vi "Get ni_measurementlink_measurement_v1_GetMetadataResponse.vi"(8 "error in (no error)":errorcluster, 11 "gRPCid":T1) -> (0 "error out":errorcluster, 2 "package_templatemessage":T2, 3 "gRPCid out":T1)   [LabVIEW 2020, in "MeasurementLink Measurement Server Internal.lvlib"]
uses:
  MeasurementLink Measurement Server Internal.lvlib
  ni_measurementlink_measurement_v1_GetMetadataResponse.ctl
  ni_measurementlink_measurement_v1_MeasurementDetails.ctl
  ni_measurementlink_measurement_v1_MeasurementSignature.ctl
  ni_measurementlink_measurement_v1_ConfigurationParameter.ctl
  google_protobuf_Field_Kind.ctl
  ni_measurementlink_measurement_v1_ConfigurationParameter_AnnotationsEntry.ctl
  google_protobuf_Any.ctl
  ni_measurementlink_measurement_v1_Output.ctl
  ni_measurementlink_measurement_v1_UserInterfaceDetails.ctl
  <vilib>/gRPC/LabVIEW gRPC Library/Shared/grpcId.ctl
  ni_measurementlink_measurement_v1_GetMetadataResponse_Flat.ctl
  ni_measurementlink_measurement_v1_MeasurementDetails_Flat.ctl
  ni_measurementlink_measurement_v1_MeasurementSignature_Flat.ctl
  ni_measurementlink_measurement_v1_ConfigurationParameter_Flat.ctl
  ni_measurementlink_measurement_v1_ConfigurationParameter_AnnotationsEntry_Flat.ctl
  google_protobuf_Any_Flat.ctl
  ni_measurementlink_measurement_v1_Output_Flat.ctl
  ni_measurementlink_measurement_v1_UserInterfaceDetails_Flat.ctl
  2ed25e12-861d-4677-8ead-ace2906b2041.vi
  <vilib>/gRPC/LabVIEW gRPC Library/Shared/TranslateGrpcError.vi
  FlatToRichni_measurementlink_measurement_v1_MeasurementDetails.vi
  FlatToRichni_measurementlink_measurement_v1_MeasurementSignature.vi
  FlatToRichni_measurementlink_measurement_v1_UserInterfaceDetails.vi
  FlatToRichni_measurementlink_measurement_v1_ConfigurationParameter.vi
  FlatToRichgoogle_protobuf_Any.vi
  FlatToRichni_measurementlink_measurement_v1_Output.vi
  FlatToRichni_measurementlink_measurement_v1_ConfigurationParameter_AnnotationsEntry.vi
  <vilib>/gRPC/LabVIEW gRPC Library/Server API/Server/Get Server DLL Path.vi
  <vilib>/Utility/error.llb/Error Cluster From Error Code.vi
  <vilib>/Utility/error.llb/Simple Error Handler.vi
  <vilib>/gRPC/LabVIEW gRPC Library/grpc-lvsupport-release.lvlib
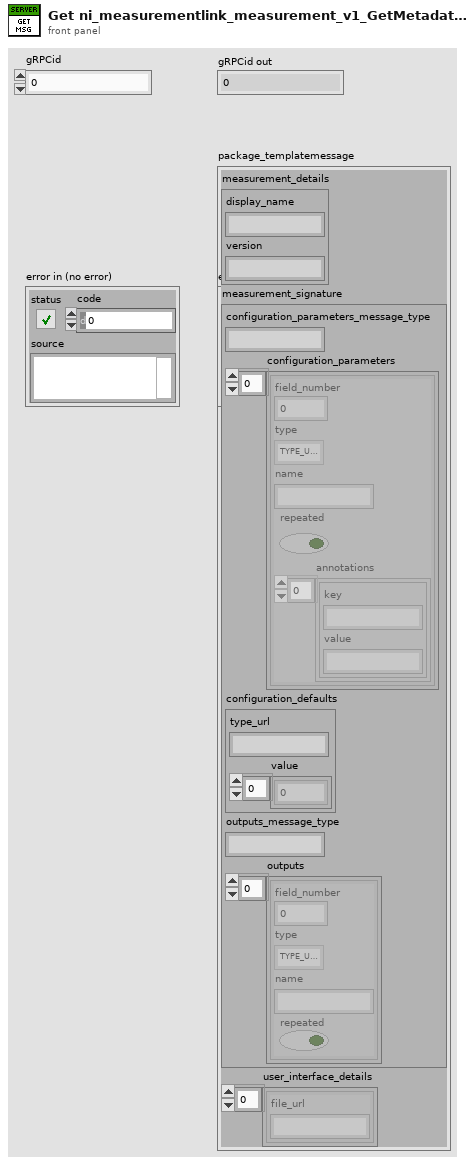
[diagram p1: front panel]
types:
  T1 = typedef "grpc-lvsupport-release.lvlib/grpcId.ctl" = u64
  T2 = typedef "MeasurementLink Measurement Server Internal.lvlib/ni_measurementlink_measurement_v1_GetMetadataResponse.ctl" = cluster{"measurement_details":T3, "measurement_signature":T4, "user_interface_details":T10[]}
  T3 = typedef "MeasurementLink Measurement Server Internal.lvlib/ni_measurementlink_measurement_v1_MeasurementDetails.ctl" = cluster{"display_name":string, "version":string}
  T4 = typedef "MeasurementLink Measurement Server Internal.lvlib/ni_measurementlink_measurement_v1_MeasurementSignature.ctl" = cluster{"configuration_parameters_message_type":string, "configuration_parameters":T5[], "configuration_defaults":T8, "outputs_message_type":string, "outputs":T9[]}
  T5 = typedef "MeasurementLink Measurement Server Internal.lvlib/ni_measurementlink_measurement_v1_ConfigurationParameter.ctl" = cluster{"field_number":i32, "type":T6, "name":string, "repeated":bool, "annotations":T7[]}
  T6 = typedef "MeasurementLink Measurement Server Internal.lvlib/google_protobuf_Field_Kind.ctl" = enum32{"TYPE_UNKNOWN", "TYPE_DOUBLE", "TYPE_FLOAT", "TYPE_INT64", "TYPE_UINT64", "TYPE_INT32", "TYPE_FIXED64", "TYPE_FIXED32", "TYPE_BOOL", "TYPE_STRING", "TYPE_GROUP", "TYPE_MESSAGE", "TYPE_BYTES", "TYPE_UINT32", "TYPE_ENUM", "TYPE_SFIXED32", "TYPE_SFIXED64", "TYPE_SINT32", "TYPE_SINT64"}
  T7 = typedef "MeasurementLink Measurement Server Internal.lvlib/ni_measurementlink_measurement_v1_ConfigurationParameter_AnnotationsEntry.ctl" = cluster{"key":string, "value":string}
  T8 = typedef "MeasurementLink Measurement Server Internal.lvlib/google_protobuf_Any.ctl" = cluster{"type_url":string, "value":u8[]}
  T9 = typedef "MeasurementLink Measurement Server Internal.lvlib/ni_measurementlink_measurement_v1_Output.ctl" = cluster{"field_number":i32, "type":T6, "name":string, "repeated":bool}
  T10 = typedef "MeasurementLink Measurement Server Internal.lvlib/ni_measurementlink_measurement_v1_UserInterfaceDetails.ctl" = cluster{"file_url":string}
  T11 = typedef "MeasurementLink Measurement Server Internal.lvlib/ni_measurementlink_measurement_v1_GetMetadataResponse_Flat.ctl" = cluster{"measurement_details":T12, "measurement_signature":T13, "user_interface_details":T18[]}
  T12 = typedef "MeasurementLink Measurement Server Internal.lvlib/ni_measurementlink_measurement_v1_MeasurementDetails_Flat.ctl" = cluster{"display_name":string, "version":string}
  T13 = typedef "MeasurementLink Measurement Server Internal.lvlib/ni_measurementlink_measurement_v1_MeasurementSignature_Flat.ctl" = cluster{"configuration_parameters_message_type":string, "configuration_parameters":T14[], "configuration_defaults":T16, "outputs_message_type":string, "outputs":T17[]}
  T14 = typedef "MeasurementLink Measurement Server Internal.lvlib/ni_measurementlink_measurement_v1_ConfigurationParameter_Flat.ctl" = cluster{"field_number":i32, "type":T6, "name":string, "repeated":bool, "annotations":T15[]}
  T15 = typedef "MeasurementLink Measurement Server Internal.lvlib/ni_measurementlink_measurement_v1_ConfigurationParameter_AnnotationsEntry_Flat.ctl" = cluster{"key":string, "value":string}
  T16 = typedef "MeasurementLink Measurement Server Internal.lvlib/google_protobuf_Any_Flat.ctl" = cluster{"type_url":string, "value":u8[]}
  T17 = typedef "MeasurementLink Measurement Server Internal.lvlib/ni_measurementlink_measurement_v1_Output_Flat.ctl" = cluster{"field_number":i32, "type":T6, "name":string, "repeated":bool}
  T18 = typedef "MeasurementLink Measurement Server Internal.lvlib/ni_measurementlink_measurement_v1_UserInterfaceDetails_Flat.ctl" = cluster{"file_url":string}
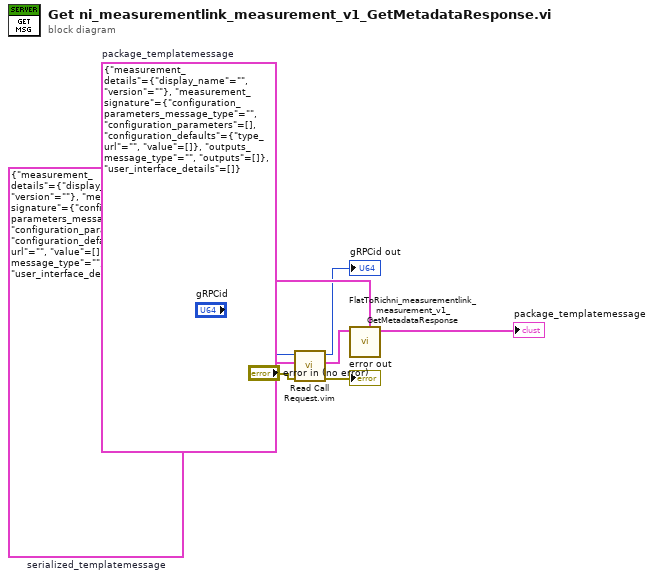
[diagram p0: block diagram]
diagram:
  w6 = T11 {"measurement_details"={"display_name"="", "version"=""}, "measurement_signature"={"configuration_parameters_message_type"="", "configuration_parameters"=[], "configuration_defaults"={"type_url"="", "value"=[]}, "outputs_message_type"="", "outputs"=[]}, "user_interface_details"=[]}  # serialized_templatemessage
  w5 = T2 {"measurement_details"={"display_name"="", "version"=""}, "measurement_signature"={"configuration_parameters_message_type"="", "configuration_parameters"=[], "configuration_defaults"={"type_url"="", "value"=[]}, "outputs_message_type"="", "outputs"=[]}, "user_interface_details"=[]}  # package_templatemessage
  n1 = call "Read Call Request.vim"("error in"="error in (no error)", "Request Type"=w6, "gRPCid in"="gRPCid") -> ("error out"=→"error out":errorcluster, "Request Data"=w4:T11, "gRPCid out"=→"gRPCid out":T1)  [unwired: 6 in]
  n2 = call "FlatToRichni_measurementlink_measurement_v1_GetMetadataResponse.vi"("OutputClusterType"=w5, "InputCluster"=w4) -> ("OutputCluster"=→"package_templatemessage":T2)  [unwired: 9 in]
